vi "Set Width.vi"(8 "error in":errorcluster, 10 "Width":i32, 11 "Generic Image in":refnum<class "Generic Image.lvclass">) -> (0 "error out":errorcluster, 3 "Generic Image out":refnum<class "Generic Image.lvclass">)   [LabVIEW 2019, in "Generic Image.lvclass"]
uses:
  Generic Image.lvclass
  Generic Image.lvclass/Generic Image.ctl
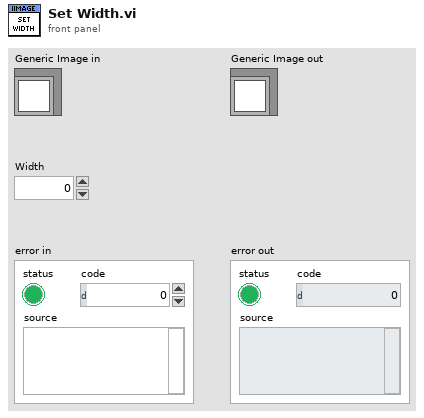
[diagram p1: front panel]
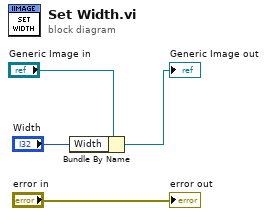
[diagram p0: block diagram]
diagram:
  n1 = Bundle By Name(cluster="Generic Image in", "Width"="Width") -> (→"Generic Image out":refnum<class "Generic Image.lvclass">)
  "error out" <- "error in"
